vi "Write acquisition configuration.vi"(8 "error in (no error)":errorcluster, 11 "Channel in":refnum<class "Channel.lvclass">) -> (0 "error out":errorcluster, 3 "Channel out":refnum<class "Channel.lvclass">)   [LabVIEW 2018, in "Channel.lvclass"]
uses:
  Channel.lvclass
  Channel.lvclass/Channel.ctl
  Simulated_CCD_Camera/Simulated Camera.lvclass
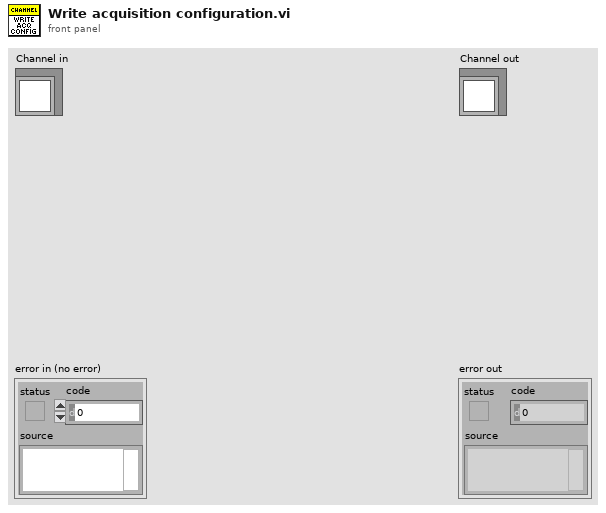
[diagram p1: front panel]
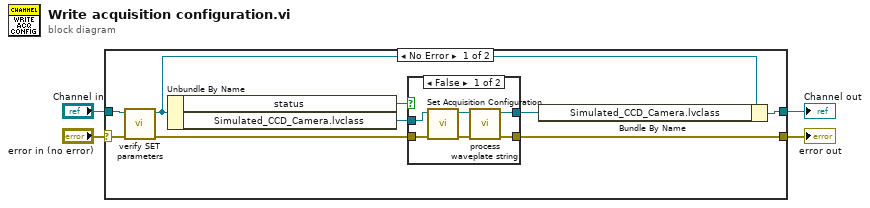
[diagram p0: block diagram]
diagram:
  n1 = case shown="No Error" "error in (no error)" {
    selector: "error in (no error)" -> [w7 w23]
    tunnel: [w10 w23] -> w3
    tunnel: [w5 w22] -> w1
    tunnel: "Channel in" -> [w6 w22]
    frame No Error {
      n2 = call "verify SET parameters.vi"("error in (no error)"=w7, "Channel in"=w6) -> ("error out"=w8:errorcluster, "Channel out"=w9:refnum<class "Channel.lvclass">)  [unwired: 8 in]
      n3 = Unbundle By Name(w9) -> ("status"=w13:bool, "Simulated_CCD_Camera.lvclass"=w12:refnum<class "Simulated Camera.lvclass">)
      n4 = case shown="False" w13 {
        tunnel: w12 -> [w18 w21]
        tunnel: w8 -> [w19 w20]
        tunnel: [w17 w20] -> w10
        tunnel: [w16 w21] -> w11
        frame False {
          n5 = call-dynamic "Set Acquisition Configuration.vi"("error in (no error)"=w19, "CCDCamera in"=w18) -> ("error out"=w14:errorcluster, "CCDCamera out"=w15:refnum<class "Simulated Camera.lvclass">)  [unwired: 8 in]
          n6 = call "process waveplate string.vi"("error in (no error)"=w14, "Simulated_CCD_Camera in"=w15) -> ("error out"=w17:errorcluster, "Simulated_CCD_Camera out"=w16:refnum<class "Simulated Camera.lvclass">)  [unwired: 8 in]
        }
        frame True {
        }
      }
      n7 = Bundle By Name(cluster=w9, "Simulated_CCD_Camera.lvclass"=w11) -> (w5:refnum<class "Channel.lvclass">)
    }
    frame Error {
    }
  }
  "error out" <- w3
  "Channel out" <- w1
